vi "Automatic-Approach-Retraction-MCL-2013-04-28-1a-data-storage-1b1-Aidan's Version-to-play-with.vi"() -> ()   [LabVIEW 2012]
uses:
  <vilib>/rvi/eio/common/nirviEmuTemplateMethod_errors.vi
  <vilib>/rvi/Emulation/niFpgaSctlEmulationGetInTimedLoop.vi
  <vilib>/rvi/Emulation/niFpgaSctlEmulationGlobalWrite.vi
  <vilib>/rvi/interface/RandomDataEmulation/nirviRandomDataFPGAFIFO.vi
  <vilib>/rvi/interface/RandomDataEmulation/niFpgaRandomDataHandleErrors.vi
  <vilib>/eio/EIONode/EIONode.xnode
  <vilib>/rvi/DataTransferAndStorage/Container/XNode/niFpgaContainer.xnode
  <vilib>/rvi/interface/RandomDataEmulation/nirviRandomDataFpgaReadWriteTemplate.vi
  <vilib>/rvi/Analysis/measure/butterworth/XNode/niFpgaButterworthFilter.xnode
panel:
  out "TF-drift":i16
  out "Tick Count(Ticks)":u32=3198398528
  in  "Data Acquisition Rate (usec)":u32=500000
  out "Data storage":bool=TRUE
  out "Start Approach indicator":bool
  in  "safetip time wait":u32 caption="Count(uSec)"
  out "safetip minimum indicator":bool
  out "Data counter":u16
  out "Counter Output":i16
  in  "Initial Position":i16
  in  "phase 1 control":bool
  in  "Manual Control":bool
  in  "Zposition MCL fine 2":i16
  in  "MCL counter 2":u16
  out "Curve indicator":u16
  in  "Number of curves":u16
  out "TF Freq shift":i16
  in  "Timeout FIFO":i32=-1
  in  "Safetip Minimum":i16
  out "Phase 2":bool
  in  "Parameter":i16
  out "Phase 1":bool
  in  "Start Approach":bool
  out "MCL counter in range?":bool
  in  "Wait-tip-before-new-approach (usec)":u32
  in  "Fast Retraction After Cycle":i32
  in  "Wait-tip-before-approach":u32
  in  "Fast Retraction before approach":i32
  in  "Offset for Fast Approach":i16
  in  "Fast Approach (usec)":u32
  in  "Minimum for Approach Value":i16
  out "digital steps per region":u16
  in  "MCL Divisions":u16
  in  "MCL counter":u16
  in  "Fine Retraction (usec)":u32
  in  "TF at infinity":i16
  out "TF Phase Signal":i16(graph)
  out "Control Signal":i16
  in  "Fine Approach (usec)":u32
  in  "Setpoint Fine":i16
  out "Zposition MCL fine":i16
  in  "Initial Height (Fine)":i16=9113
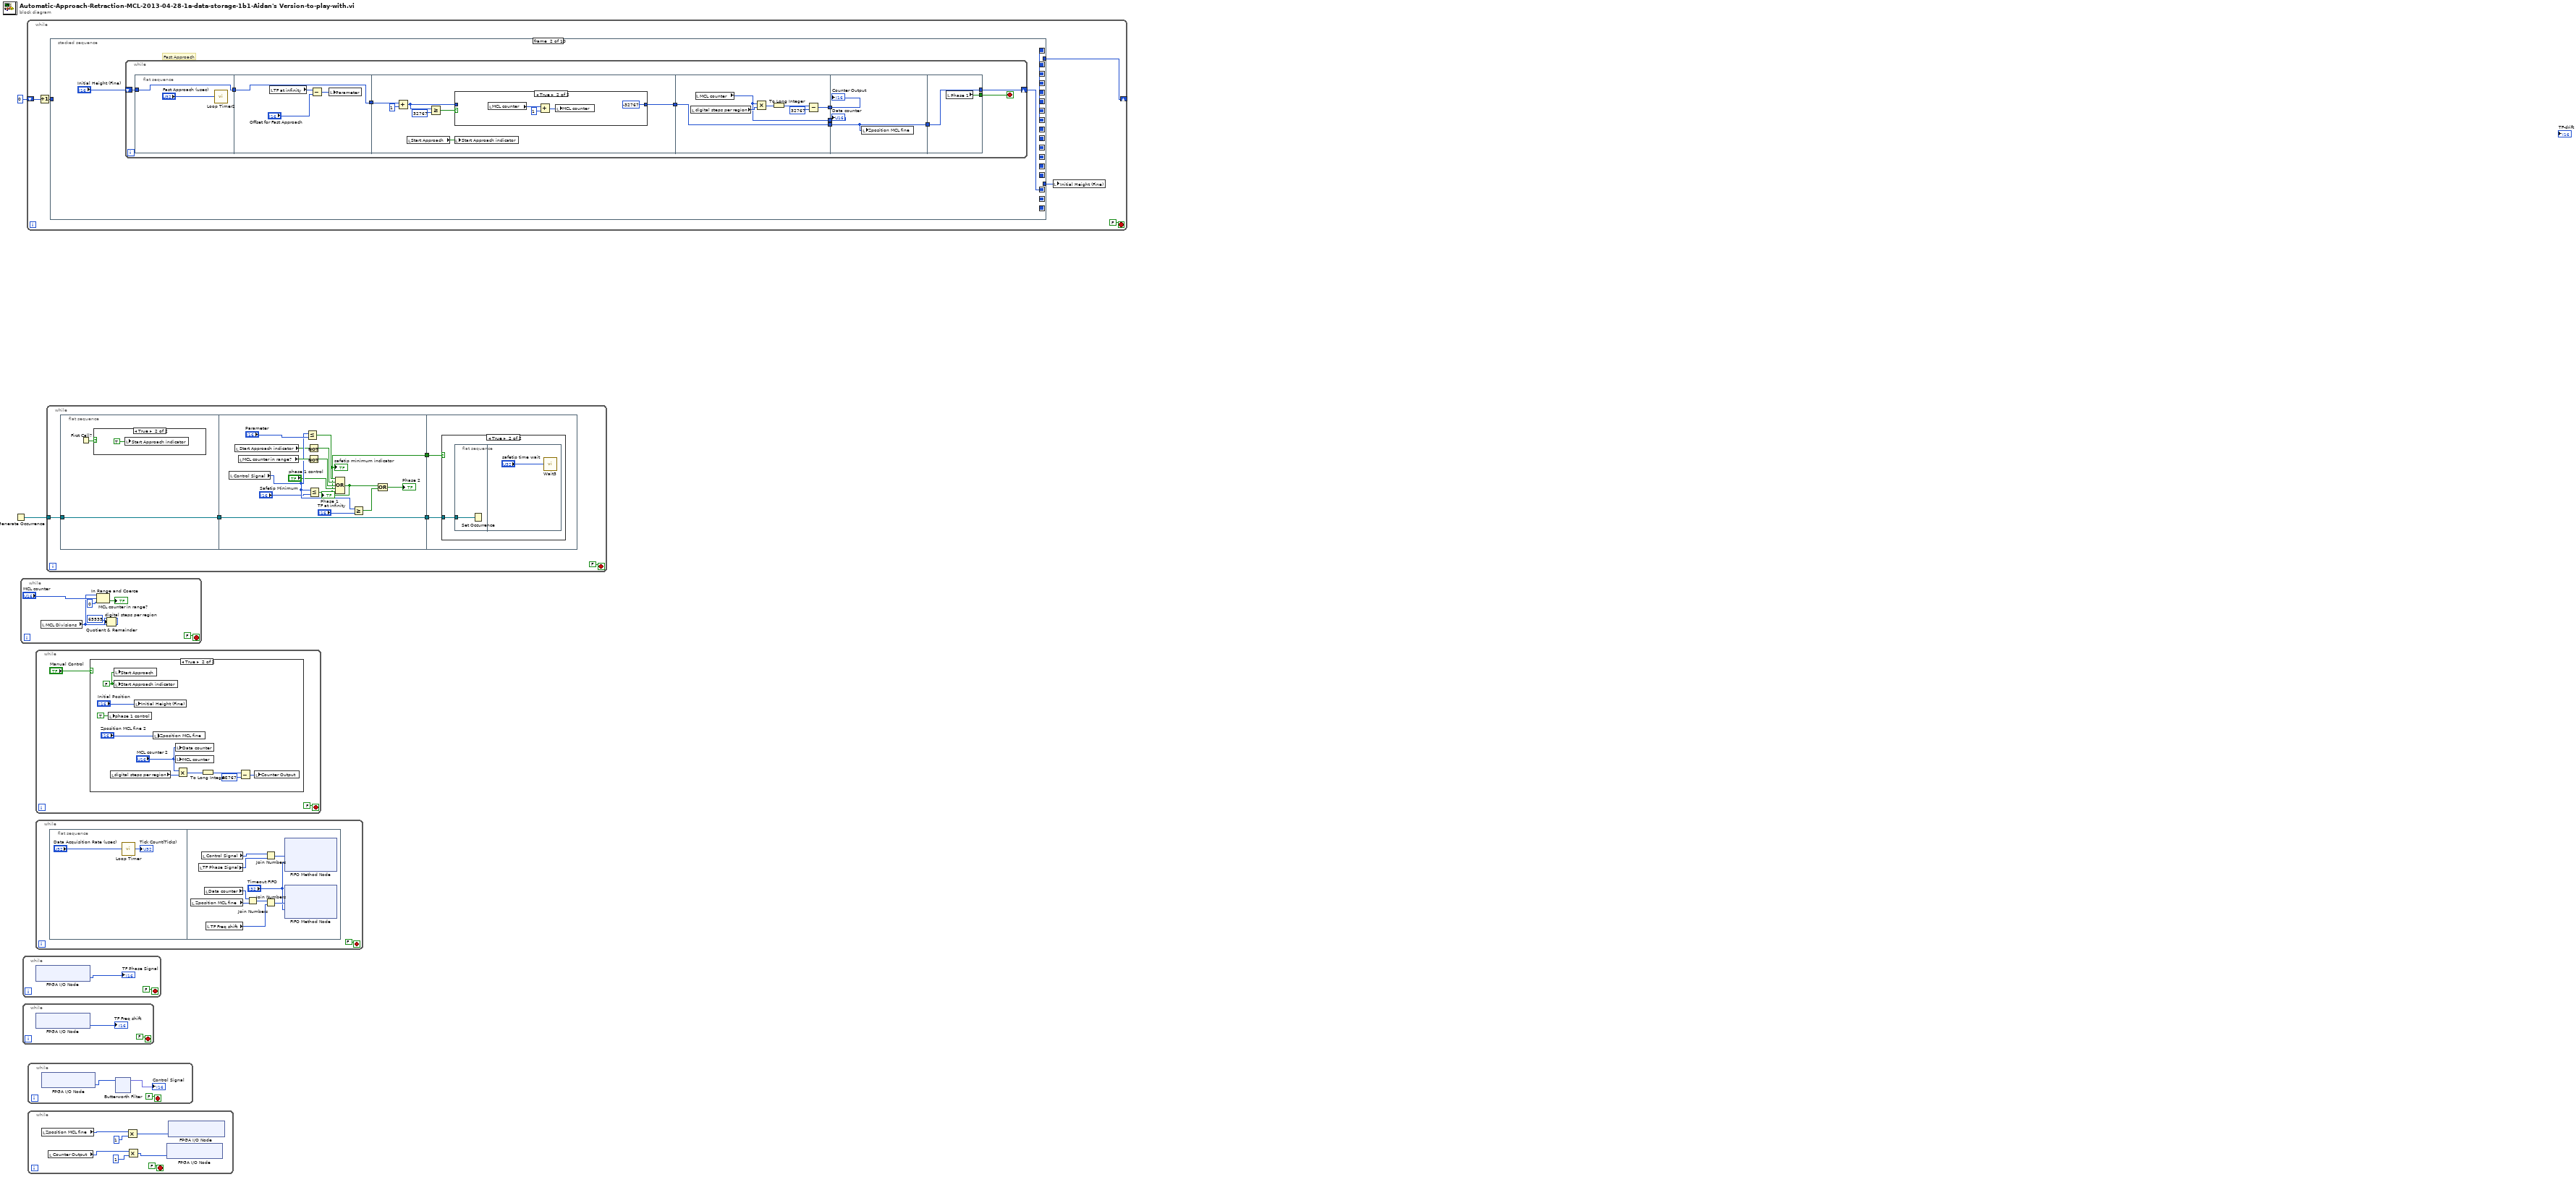
[diagram p0: block diagram]
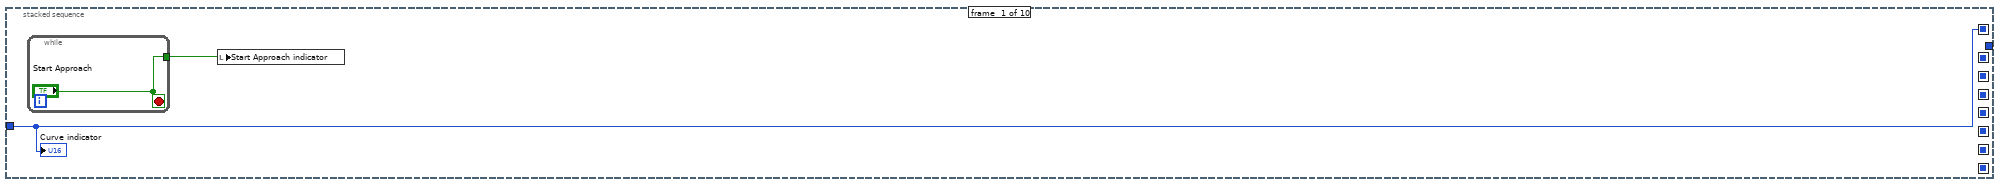
[diagram p5: hidden frame]
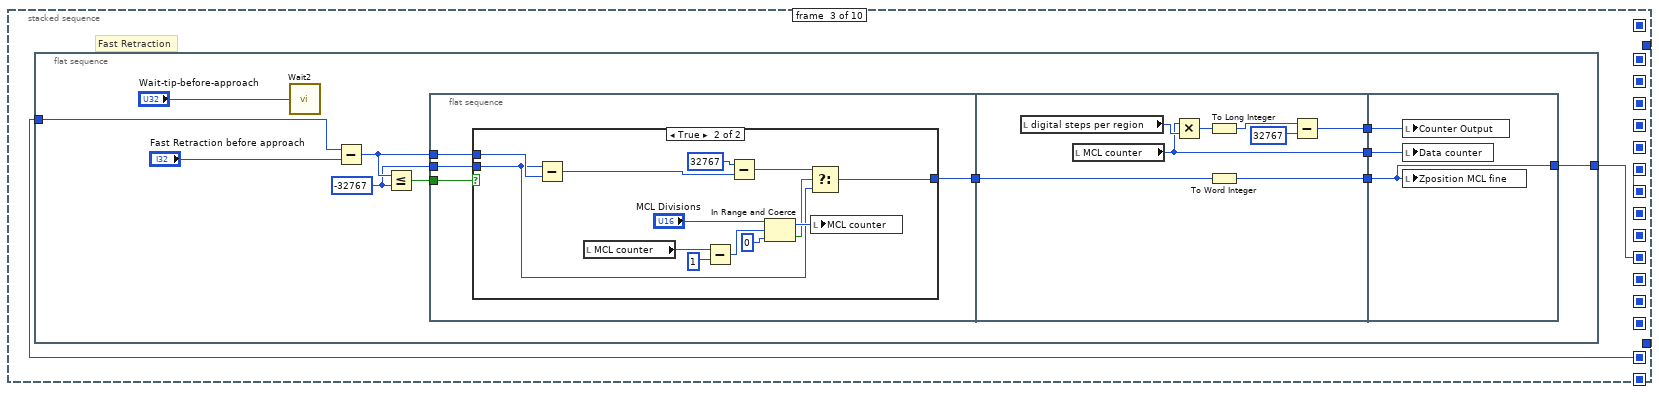
[diagram p7: hidden frame]
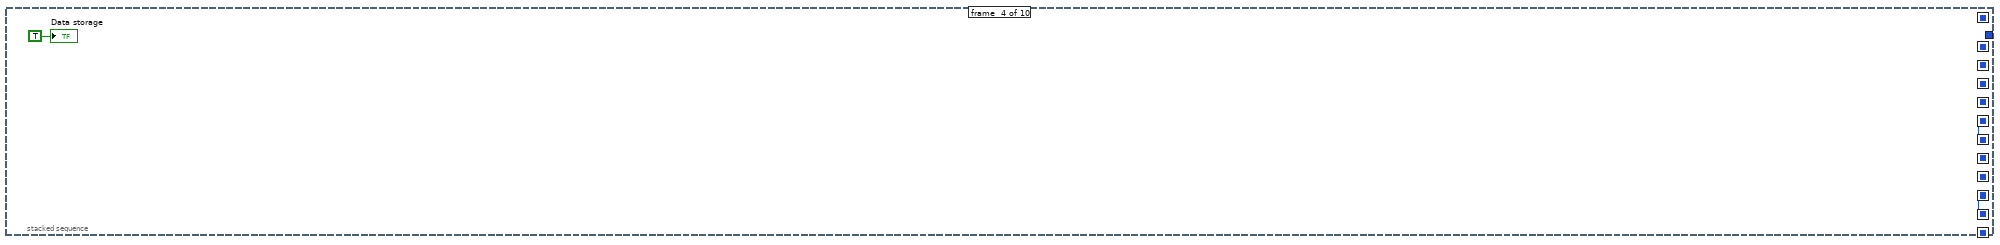
[diagram p9: hidden frame]
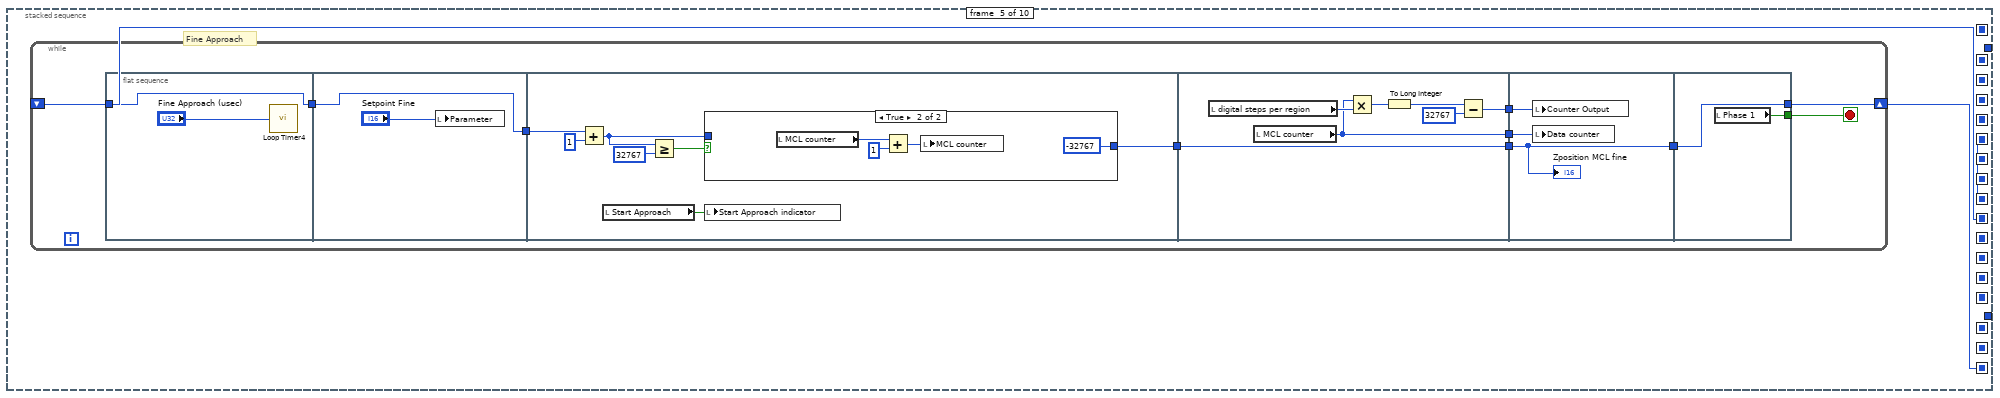
[diagram p10: hidden frame]
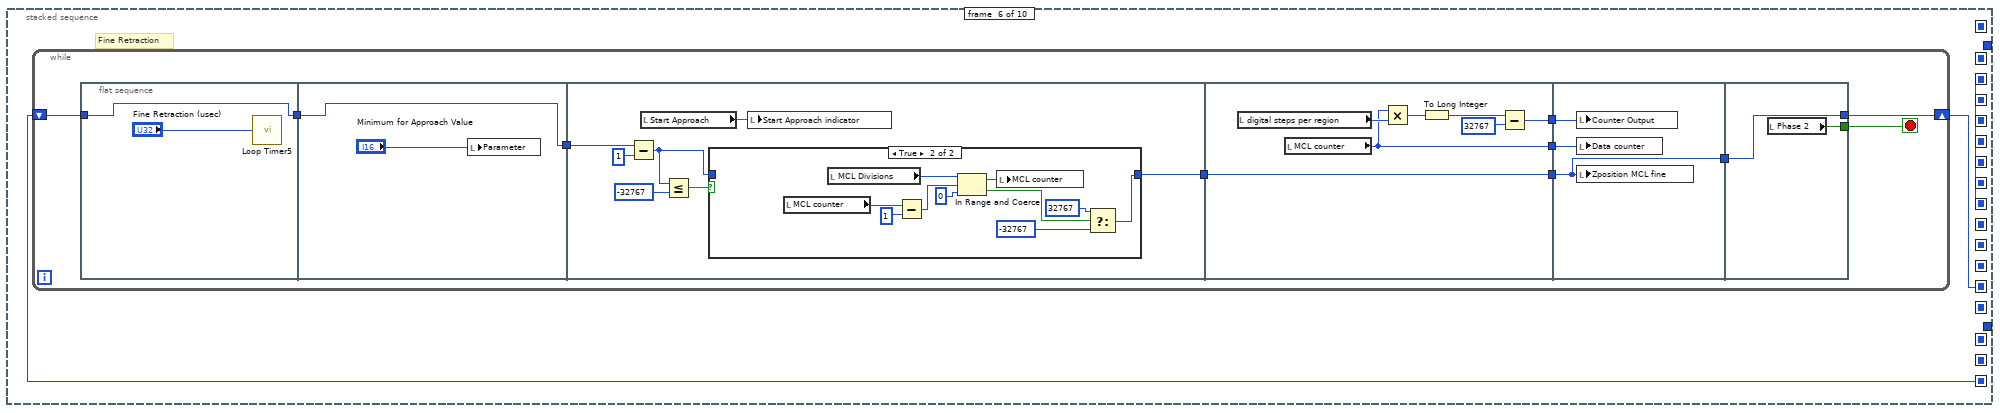
[diagram p12: hidden frame]
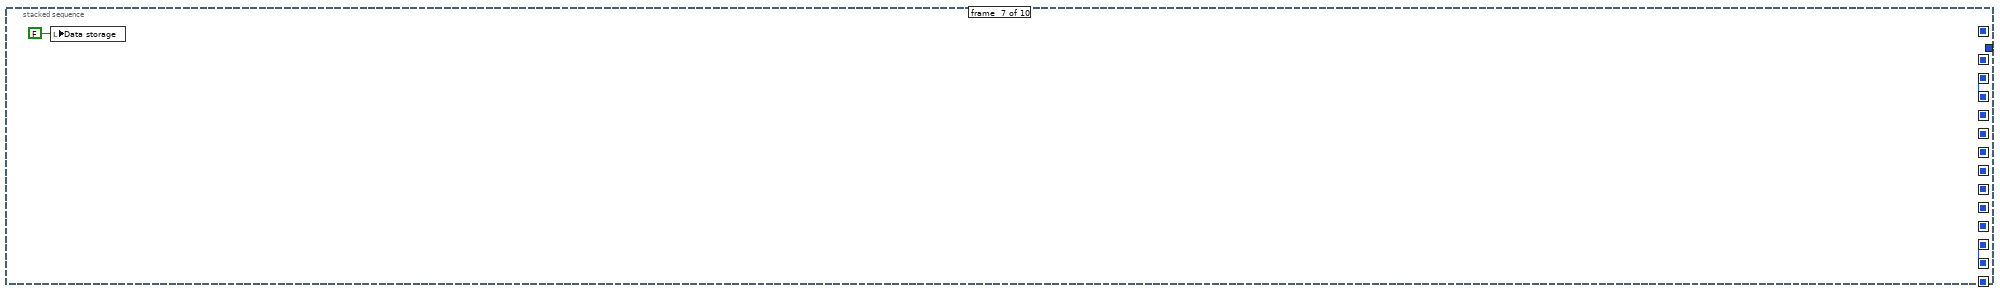
[diagram p14: hidden frame]
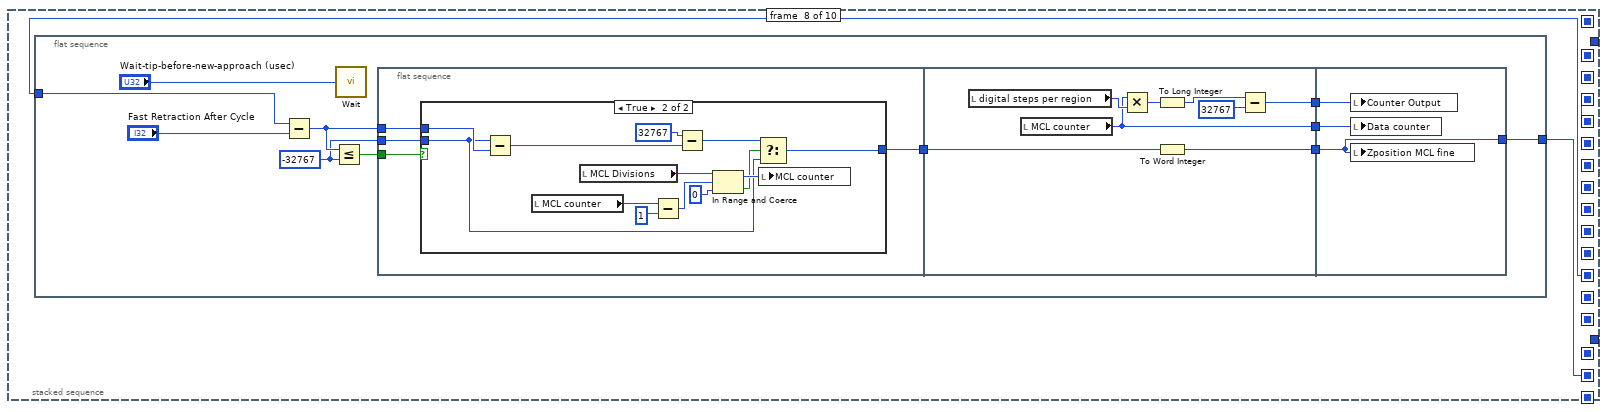
[diagram p15: hidden frame]
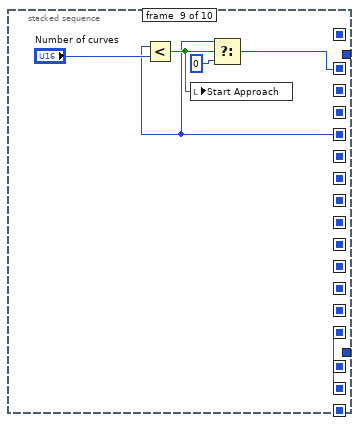
[diagram p17: hidden frame]
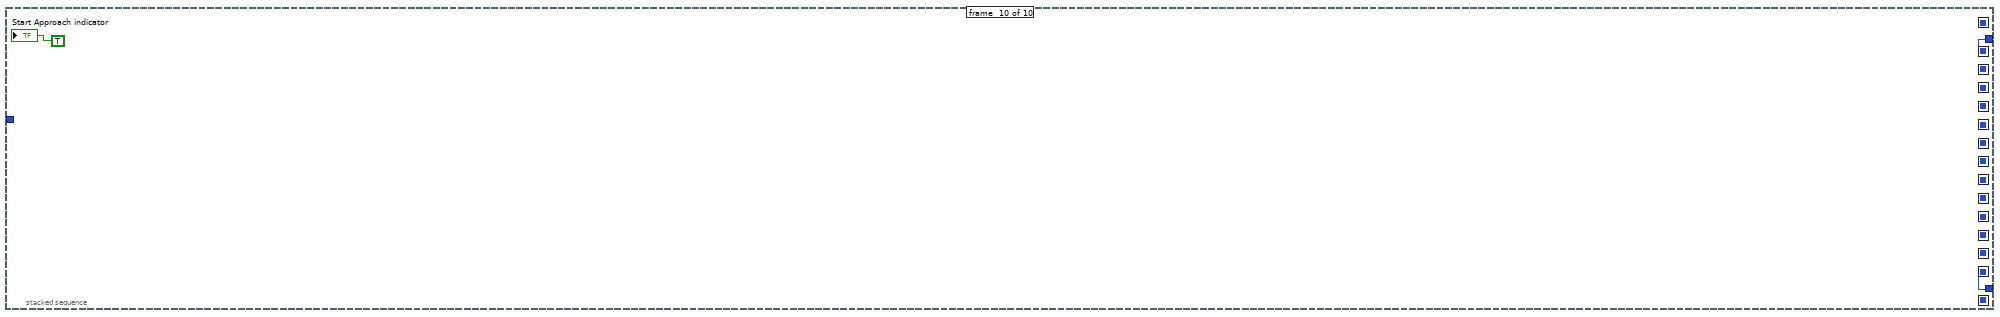
[diagram p18: hidden frame]
diagram:
  n1 = Generate Occurrence() -> (w1:refnum<k4>)
  n2 = while {
    stop <- FALSE stop-if-true
    n3 = local read "MCL Divisions"() -> (w3:u16)
    n4 = In Range and Coerce(upper limit=w3, x="MCL counter", lower limit=u16 0) -> (In Range?=→"MCL counter in range?":bool)  [unwired: 1 out]
    n5 = Quotient & Remainder(x=65535, y=w3) -> (floor(x/y)=→"digital steps per region":i32)  [unwired: 1 out]
  }
  n6 = while {
    stop <- FALSE stop-if-true
    n7 = xnode "FPGA I/O Node"() -> ("Connector0/AI1"=→"TF Phase Signal":i16)  [unwired: 1 in, 1 out]
  }
  n8 = while {
    stop <- FALSE stop-if-true
    n9 = xnode "FPGA I/O Node"() -> ("Connector0/AI2"=→"TF Freq shift":i16)  [unwired: 1 in, 1 out]
  }
  n10 = while {
    shift-right: [w15] -> _
    shift-left: u16 0 ("t") -> [w14]
    stop <- FALSE stop-if-true
    n11 = Increment(x=w14) -> (x+1=w16:u16)
    n12 = stacked-sequence {
      seq-local: [w20 _ _ _ _ _ _ _ _ _] -> [_ w23 _ _ _ _ _ _ _ _]
      seq-local: [_ w24 _ _ _ _ _ _ _ _] -> [_ _ w67 _ _ _ _ _ _ _]
      seq-local: [_ w23 _ _ _ _ _ _ _ _] -> [_ _ w65 _ _ _ _ _ _ _]
      seq-local: [_ _ w66 _ _ _ _ _ _ _] -> [_ _ _ w110 _ _ _ _ _ _]
      seq-local: [_ _ w65 _ _ _ _ _ _ _] -> [_ _ _ w109 _ _ _ _ _ _]
      seq-local: [_ _ _ w110 _ _ _ _ _ _] -> [_ _ _ _ w113 _ _ _ _ _]
      seq-local: [_ _ _ w109 _ _ _ _ _ _] -> [_ _ _ _ w111 _ _ _ _ _]
      seq-local: [_ _ _ _ w112 _ _ _ _ _] -> [_ _ _ _ _ w154 _ _ _ _]
      seq-local: [_ _ _ _ w111 _ _ _ _ _] -> [_ _ _ _ _ w152 _ _ _ _]
      seq-local: [_ _ _ _ _ w153 _ _ _ _] -> [_ _ _ _ _ _ w201 _ _ _]
      seq-local: [_ _ _ _ _ w152 _ _ _ _] -> [_ _ _ _ _ _ w200 _ _ _]
      seq-local: [_ _ _ _ _ _ w201 _ _ _] -> [_ _ _ _ _ _ _ w204 _ _]
      seq-local: [_ _ _ _ _ _ w200 _ _ _] -> [_ _ _ _ _ _ _ w202 _ _]
      seq-local: [_ _ _ _ _ _ _ w203 _ _] -> [_ _ _ _ _ _ _ _ w250 _]
      seq-local: [_ _ _ _ _ _ _ w202 _ _] -> [_ _ _ _ _ _ _ _ w245 _]
      seq-local: [_ _ _ _ _ _ _ _ w250 _] -> [_ _ _ _ _ _ _ _ _ w253]
      seq-local: [_ _ _ _ _ _ _ _ w246 _] -> [_ _ _ _ _ _ _ _ _ w252]
      tunnel: w16 -> [w20 _ _ _ _ _ _ _ _ _]
      tunnel: [_ _ _ _ _ _ _ _ _ w253] -> w18
      tunnel: [_ _ _ _ _ _ _ _ _ w252] -> w15
      frame #0 {
        n13 = while {
          tunnel: ["Start Approach"] -> w19
          stop <- "Start Approach" stop-if-true
        }
        n14 = local write "Start Approach indicator"(w19) -> ()
        "Curve indicator" <- w20
      }
      frame #1 {
        # "Fast Approach"
        n15 = while {
          shift-right: [w33] -> w24
          shift-left: "Initial Height (Fine)" -> [w34]
          stop <- w29 stop-if-true
          n16 = flat-sequence {
            tunnel: w34 -> [w36]
            tunnel: [w36] -> w31
            tunnel: [w40] -> w32
            tunnel: w31 -> [w40]
            tunnel: [w46] -> w28
            tunnel: w32 -> [w47]
            tunnel: w28 -> [w59]
            tunnel: [w59] -> w27
            tunnel: [w56] -> w26
            tunnel: [w55] -> w25
            tunnel: w27 -> [w62]
            tunnel: [w62] -> w30
            tunnel: w26 -> [w61]
            tunnel: w25 -> [w60]
            tunnel: [w64] -> w33
            tunnel: w30 -> [w64]
            tunnel: [w63] -> w29
            frame #0 {
              n17 = call "Loop Timer2"("Count(uSec)"="Fast Approach (usec)") -> ()  [unwired: 1 out]
            }
            frame #1 {
              n18 = local read "TF at infinity"() -> (w37:i16)
              n19 = Subtract(x=w37, y="Offset for Fast Approach") -> (x-y=w39:i16)
              n20 = local write "Parameter"(w39) -> ()
            }
            frame #2 {
              n21 = Add(x=w47, y=i16 1) -> (x+y=w42:i16)
              n22 = local read "Start Approach"() -> (w41:bool)
              n23 = Greater Or Equal?(x=w42, y=i16 32767) -> (x >= y?=w43:bool)
              n24 = case shown="True" w43 {
                tunnel: [w48 i16 -32767] -> w46
                tunnel: w42 -> [w48 _]
                frame False {
                }
                frame True {
                  n25 = local read "MCL counter"() -> (w50:u16)
                  n26 = Add(x=w50, y=u16 1) -> (x+y=w49:u16)
                  n27 = local write "MCL counter"(w49) -> ()
                }
              }
              n28 = local write "Start Approach indicator"(w41) -> ()
            }
            frame #3 {
              n29 = local read "digital steps per region"() -> (w58:u16)
              n30 = local read "MCL counter"() -> (w55:u16)
              n31 = Multiply(x=w55, y=w58) -> (x*y=w54:u16)
              n32 = To Long Integer(number=w54) -> (32bit integer=w53:i32)
              n33 = Subtract(x=w53, y=32767) -> (x-y=w56:i32)
            }
            frame #4 {
              n34 = local write "Zposition MCL fine"(w62) -> ()
              "Counter Output" <- w61
              "Data counter" <- w60
            }
            frame #5 {
              n35 = local read "Phase 1"() -> (w63:bool)
            }
          }
        }
      }
      frame #2 {
        # "Fast Retraction"
        n36 = flat-sequence {
          tunnel: [w74] -> w66
          tunnel: w67 -> [w75]
          frame #0 {
            w72 = -32767 ("y")
            n37 = call "Wait2"("Count(uSec)"="Wait-tip-before-approach") -> ()  [unwired: 1 out]
            n38 = Subtract(x=w75, y="Fast Retraction before approach") -> (x-y=w77:i32)
            n39 = Less Or Equal?(x=w77, y=w72) -> (x <= y?=w78:bool)
            n40 = flat-sequence {
              tunnel: w78 -> [w82]
              tunnel: w77 -> [w81]
              tunnel: w72 -> [w79]
              tunnel: [w80] -> w71
              tunnel: w71 -> [w100]
              tunnel: [w99] -> w70
              tunnel: [w101] -> w69
              tunnel: [w102] -> w68
              tunnel: [w107] -> w74
              tunnel: w70 -> [w107]
              tunnel: w69 -> [w106]
              tunnel: w68 -> [w105]
              frame #0 {
                n41 = case shown="True" w82 {
                  tunnel: w81 -> [w83 w93]
                  tunnel: [w83 w85] -> w80
                  tunnel: w79 -> [_ w84]
                  frame False {
                  }
                  frame True {
                    n42 = Subtract(x=w84, y=w93) -> (x-y=w92:i32)
                    n43 = local read "MCL counter"() -> (w96:u16)
                    n44 = Subtract(x=w96, y=u16 1) -> (x-y=w89:u16)
                    n45 = Subtract(x=32767, y=w92) -> (x-y=w86:i32)
                    n46 = In Range and Coerce(upper limit="MCL Divisions", x=w89, lower limit=u16 0 ("upper limit")) -> (coerced(x)=w88:u16, In Range?=w87:bool)
                    n47 = Select(t=w86, s=w87, f=w84) -> (s? t:f=w85:i32)
                    n48 = local write "MCL counter"(w88) -> ()
                  }
                }
              }
              frame #1 {
                n49 = local read "digital steps per region"() -> (w104:u16)
                n50 = local read "MCL counter"() -> (w101:u16)
                n51 = Multiply(x=w101, y=w104) -> (x*y=w98:u16)
                n52 = To Long Integer(number=w98) -> (32bit integer=w97:i32)
                n53 = To Word Integer(number=w100) -> (16bit integer=w99:i16)
                n54 = Subtract(x=w97, y=32767) -> (x-y=w102:i32)
              }
              frame #2 {
                n55 = local write "Counter Output"(w105) -> ()
                n56 = local write "Data counter"(w106) -> ()
                n57 = local write "Zposition MCL fine"(w107) -> ()
              }
            }
          }
        }
      }
      frame #3 {
        "Data storage" <- TRUE
      }
      frame #4 {
        # "Fine Approach"
        n58 = while {
          shift-right: [w122] -> w112
          shift-left: w113 -> [w123]
          stop <- w114 stop-if-true
          n59 = flat-sequence {
            tunnel: w123 -> [w125]
            tunnel: [w125] -> w120
            tunnel: [w127] -> w121
            tunnel: w120 -> [w127]
            tunnel: [w133] -> w119
            tunnel: w121 -> [w134]
            tunnel: w119 -> [w146]
            tunnel: [w146] -> w118
            tunnel: [w143] -> w117
            tunnel: [w142] -> w116
            tunnel: w118 -> [w147]
            tunnel: w117 -> [w149]
            tunnel: w116 -> [w148]
            tunnel: [w147] -> w115
            tunnel: [w151] -> w122
            tunnel: w115 -> [w151]
            tunnel: [w150] -> w114
            frame #0 {
              n60 = call "Loop Timer4"("Count(uSec)"="Fine Approach (usec)") -> ()  [unwired: 1 out]
            }
            frame #1 {
              n61 = local write "Parameter"("Setpoint Fine") -> ()
            }
            frame #2 {
              n62 = Add(x=w134, y=i16 1) -> (x+y=w129:i16)
              n63 = local read "Start Approach"() -> (w128:bool)
              n64 = Greater Or Equal?(x=w129, y=i16 32767) -> (x >= y?=w130:bool)
              n65 = case shown="True" w130 {
                tunnel: [w135 i16 -32767] -> w133
                tunnel: w129 -> [w135 _]
                frame False {
                }
                frame True {
                  n66 = local read "MCL counter"() -> (w136:u16)
                  n67 = Add(x=w136, y=u16 1) -> (x+y=w138:u16)
                  n68 = local write "MCL counter"(w138) -> ()
                }
              }
              n69 = local write "Start Approach indicator"(w128) -> ()
            }
            frame #3 {
              n70 = local read "digital steps per region"() -> (w145:u16)
              n71 = local read "MCL counter"() -> (w142:u16)
              n72 = Multiply(x=w142, y=w145) -> (x*y=w141:u16)
              n73 = To Long Integer(number=w141) -> (32bit integer=w140:i32)
              n74 = Subtract(x=w140, y=32767) -> (x-y=w143:i32)
            }
            frame #4 {
              n75 = local write "Counter Output"(w149) -> ()
              n76 = local write "Data counter"(w148) -> ()
              "Zposition MCL fine" <- w147
            }
            frame #5 {
              n77 = local read "Phase 1"() -> (w150:bool)
            }
          }
        }
      }
      frame #5 {
        # "Fine Retraction"
        n78 = while {
          shift-right: [w163] -> w153
          shift-left: w154 -> [w164]
          stop <- w157 stop-if-true
          n79 = flat-sequence {
            tunnel: w164 -> [w166]
            tunnel: [w166] -> w160
            tunnel: [w168] -> w161
            tunnel: w160 -> [w168]
            tunnel: [w174] -> w162
            tunnel: w161 -> [w175]
            tunnel: w162 -> [w193]
            tunnel: [w193] -> w159
            tunnel: [w188] -> w156
            tunnel: [w187] -> w155
            tunnel: w159 -> [w194]
            tunnel: [w194] -> w158
            tunnel: w156 -> [w196]
            tunnel: w155 -> [w195]
            tunnel: [w198] -> w163
            tunnel: w158 -> [w198]
            tunnel: [w197] -> w157
            frame #0 {
              n80 = call "Loop Timer5"("Count(uSec)"="Fine Retraction (usec)") -> ()  [unwired: 1 out]
            }
            frame #1 {
              n81 = local write "Parameter"("Minimum for Approach Value") -> ()
            }
            frame #2 {
              n82 = Subtract(x=w175, y=i16 1) -> (x-y=w170:i16)
              n83 = local read "Start Approach"() -> (w169:bool)
              n84 = Less Or Equal?(x=w170, y=i16 -32767) -> (x <= y?=w172:bool)
              n85 = case shown="True" w172 {
                tunnel: w170 -> [w176 _]
                tunnel: [w176 w177] -> w174
                frame False {
                }
                frame True {
                  n86 = local read "MCL counter"() -> (w186:u16)
                  n87 = local read "MCL Divisions"() -> (w184:u16)
                  n88 = Subtract(x=w186, y=u16 1) -> (x-y=w182:u16)
                  n89 = In Range and Coerce(upper limit=w184, x=w182, lower limit=u16 0) -> (coerced(x)=w181:u16, In Range?=w180:bool)
                  n90 = local write "MCL counter"(w181) -> ()
                  n91 = Select(t=i16 32767, s=w180, f=i16 -32767) -> (s? t:f=w177:i16)
                }
              }
              n92 = local write "Start Approach indicator"(w169) -> ()
            }
            frame #3 {
              n93 = local read "digital steps per region"() -> (w192:u16)
              n94 = local read "MCL counter"() -> (w188:u16)
              n95 = Multiply(x=w188, y=w192) -> (x*y=w190:u16)
              n96 = To Long Integer(number=w190) -> (32bit integer=w189:i32)
              n97 = Subtract(x=w189, y=32767) -> (x-y=w187:i32)
            }
            frame #4 {
              n98 = local write "Counter Output"(w195) -> ()
              n99 = local write "Data counter"(w196) -> ()
              n100 = local write "Zposition MCL fine"(w194) -> ()
            }
            frame #5 {
              n101 = local read "Phase 2"() -> (w197:bool)
            }
          }
        }
      }
      frame #6 {
        n102 = local write "Data storage"(FALSE ("Data storage")) -> ()
      }
      frame #7 {
        n103 = flat-sequence {
          tunnel: [w211] -> w203
          tunnel: w204 -> [w212]
          frame #0 {
            w209 = -32767 ("y")
            n104 = Subtract(x=w212, y="Fast Retraction After Cycle") -> (x-y=w215:i32)
            n105 = Less Or Equal?(x=w215, y=w209) -> (x <= y?=w214:bool)
            n106 = call "Wait"("Count(uSec)"="Wait-tip-before-new-approach (usec)") -> ()  [unwired: 1 out]
            n107 = flat-sequence {
              tunnel: w215 -> [w219]
              tunnel: w214 -> [w218]
              tunnel: w209 -> [w216]
              tunnel: [w217] -> w208
              tunnel: w208 -> [w237]
              tunnel: [w236] -> w207
              tunnel: [w239] -> w206
              tunnel: [w238] -> w205
              tunnel: [w243] -> w211
              tunnel: w207 -> [w243]
              tunnel: w206 -> [w244]
              tunnel: w205 -> [w242]
              frame #0 {
                n108 = case shown="True" w218 {
                  tunnel: w219 -> [w220 w231]
                  tunnel: [w220 w221] -> w217
                  tunnel: w216 -> [_ w222]
                  frame False {
                  }
                  frame True {
                    n109 = Subtract(x=w222, y=w231) -> (x-y=w230:i32)
                    n110 = local read "MCL counter"() -> (w233:u16)
                    n111 = local read "MCL Divisions"() -> (w227:u16)
                    n112 = Subtract(x=w233, y=u16 1) -> (x-y=w228:u16)
                    n113 = Subtract(x=32767, y=w230) -> (x-y=w223:i32)
                    n114 = In Range and Coerce(upper limit=w227, x=w228, lower limit=u16 0) -> (coerced(x)=w225:u16, In Range?=w224:bool)
                    n115 = Select(t=w223, s=w224, f=w222) -> (s? t:f=w221:i32)
                    n116 = local write "MCL counter"(w225) -> ()
                  }
                }
              }
              frame #1 {
                n117 = local read "digital steps per region"() -> (w241:u16)
                n118 = local read "MCL counter"() -> (w238:u16)
                n119 = Multiply(x=w238, y=w241) -> (x*y=w235:u16)
                n120 = To Long Integer(number=w235) -> (32bit integer=w234:i32)
                n121 = To Word Integer(number=w237) -> (16bit integer=w236:i16)
                n122 = Subtract(x=w234, y=32767) -> (x-y=w239:i32)
              }
              frame #2 {
                n123 = local write "Counter Output"(w244) -> ()
                n124 = local write "Data counter"(w242) -> ()
                n125 = local write "Zposition MCL fine"(w243) -> ()
              }
            }
          }
        }
      }
      frame #8 {
        n126 = Less?(x=w245, y="Number of curves") -> (x < y?=w248:bool)
        n127 = local write "Start Approach"(w248) -> ()
        n128 = Select(t=w245, s=w248, f=u16 0 ("t")) -> (s? t:f=w246:u16)
      }
      frame #9 {
        "Start Approach indicator" <- TRUE ("Start Approach indicator")
      }
    }
    n129 = local write "Initial Height (Fine)"(w18) -> ()
  }
  n130 = while {
    stop <- FALSE stop-if-true
    n131 = xnode "FPGA I/O Node"() -> ("Connector0/AI7"=w255:i16)  [unwired: 1 in, 1 out]
    n132 = xnode "Butterworth Filter"("input data"=w255) -> ("output data"=→"Control Signal":fxp<+/-,20,20>)  [unwired: 2 in]
  }
  n133 = while {
    stop <- FALSE stop-if-true
    n134 = local read "Zposition MCL fine"() -> (w269:i16)
    n135 = local read "Counter Output"() -> (w265:i16)
    n136 = Multiply(x=w269, y=i16 1) -> (x*y=w268:i16)
    n137 = Multiply(x=w265, y=i16 1) -> (x*y=w266:i16)
    n138 = xnode "FPGA I/O Node"("Connector0/AO2"=w266) -> ()  [unwired: 1 in, 1 out]
    n139 = xnode "FPGA I/O Node"("Connector0/AO7"=w268) -> ()  [unwired: 1 in, 1 out]
  }
  n140 = while {
    stop <- FALSE stop-if-true
    n141 = case shown="True" "Manual Control" {
      frame False {
      }
      frame True {
        w273 = FALSE ("Start Approach")
        n142 = local write "phase 1 control"(TRUE ("phase 1 control")) -> ()
        n143 = local read "digital steps per region"() -> (w279:u16)
        n144 = local write "Start Approach"(w273) -> ()
        n145 = local write "Start Approach indicator"(w273) -> ()
        n146 = local write "Initial Height (Fine)"("Initial Position") -> ()
        n147 = local write "Zposition MCL fine"("Zposition MCL fine 2") -> ()
        n148 = local write "Data counter"("MCL counter 2") -> ()
        n149 = local write "MCL counter"("MCL counter 2") -> ()
        n150 = Multiply(x="MCL counter 2", y=w279) -> (x*y=w275:u16)
        n151 = To Long Integer(number=w275) -> (32bit integer=w274:i32)
        n152 = Subtract(x=w274, y=32767) -> (x-y=w277:i32)
        n153 = local write "Counter Output"(w277) -> ()
      }
    }
  }
  n154 = while {
    stop <- FALSE stop-if-true
    n155 = flat-sequence {
      frame #0 {
        n156 = call "Loop Timer"("Count(Ticks)"="Data Acquisition Rate (usec)") -> ("Tick Count(Ticks)"=→"Tick Count(Ticks)":u32)
      }
      frame #1 {
        n157 = local read "Zposition MCL fine"() -> (w292:i16)
        n158 = local read "TF Phase Signal"() -> (w287:i16)
        n159 = local read "Control Signal"() -> (w288:i16)
        n160 = local read "Data counter"() -> (w293:u16)
        n161 = local read "TF Freq shift"() -> (w286:i16)
        n162 = Join Numbers(hi=w293, lo=w292) -> ((hi.lo)=w291:u32)
        n163 = Join Numbers(hi=w288, lo=w287) -> ((hi.lo)=w294:u32)
        n164 = Join Numbers(hi=w291, lo=w286) -> ((hi.lo)=w290:u64)
        n165 = xnode ("FIFO Method Node")("Element"=w294, "Timeout"="Timeout FIFO") -> ()  [unwired: 1 in, 2 out]
        n166 = xnode ("FIFO Method Node")("Element"=w290, "Timeout"="Timeout FIFO") -> ()  [unwired: 1 in, 2 out]
      }
    }
  }
  n167 = while {
    tunnel: w1 -> [w297]
    stop <- FALSE stop-if-true
    n168 = flat-sequence {
      tunnel: [w300] -> w298
      tunnel: w297 -> [w300]
      tunnel: [w305] -> w296
      tunnel: w298 -> [w303]
      tunnel: [w303] -> w295
      tunnel: w296 -> [w319]
      tunnel: w295 -> [w318]
      frame #0 {
        n169 = First Call?() -> (First Call?: T/F=w301:bool)
        n170 = case shown="True" w301 {
          frame False {
          }
          frame True {
            n171 = local write "Start Approach indicator"(TRUE ("Start Approach indicator")) -> ()
          }
        }
      }
      frame #1 {
        n172 = local read "Control Signal"() -> (w309:i16)
        n173 = local read "Start Approach indicator"() -> (w304:bool)
        n174 = local read "MCL counter in range?"() -> (w316:bool)
        n175 = Less Or Equal?(x=w309, y="Parameter") -> (x <= y?=w314:bool)
        n176 = Not(x=w304) -> (.not. x?=w315:bool)
        n177 = Not(x=w316) -> (.not. x?=w317:bool)
        n178 = Less Or Equal?(x=w309, y="Safetip Minimum") -> (x <= y?=w305:bool)
        "safetip minimum indicator" <- w305
        n179 = Compound Arithmetic op=OR(w314, w315, w317, "phase 1 control", w305) -> (w306:bool)
        "Phase 1" <- w306
        n180 = Greater Or Equal?(x=w309, y="TF at infinity") -> (x >= y?=w311:bool)
        n181 = Compound Arithmetic op=OR(w306, w311) -> (→"Phase 2":bool)
      }
      frame #2 {
        n182 = case shown="True" w319 {
          tunnel: w318 -> [_ w320]
          frame False {
          }
          frame True {
            n183 = flat-sequence {
              tunnel: w320 -> [w321]
              frame #0 {
                n184 = Set Occurrence(w321) -> ()
              }
              frame #1 {
                n185 = call "Wait3"("Count(uSec)"="safetip time wait") -> ()  [unwired: 1 out]
              }
            }
          }
        }
      }
    }
  }
